vi "GoTo PID rápido.vi"(8 "Position":dbl[](array[numeric]), 11 "Target":dbl[](array[numeric])) -> (3 "Velocity":dbl[](array[numeric]))   [LabVIEW 2016]
uses:
  <vilib>/Analysis/coordinate.llb/2D Cartesian Coordinate Rotation (Scalar).vi
  <vilib>/addons/control/pid/pid.llb/PID (DBL).vi
  <vilib>/addons/control/pid/NI_PID_pid.lvlib
  <vilib>/Analysis/NI_AALPro.lvlib
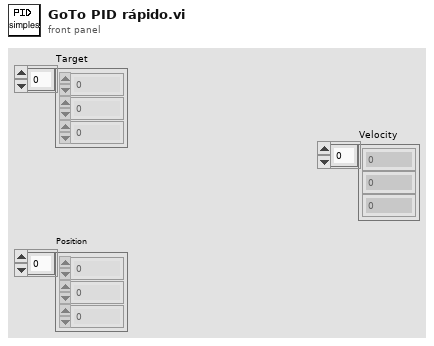
[diagram p1: front panel]
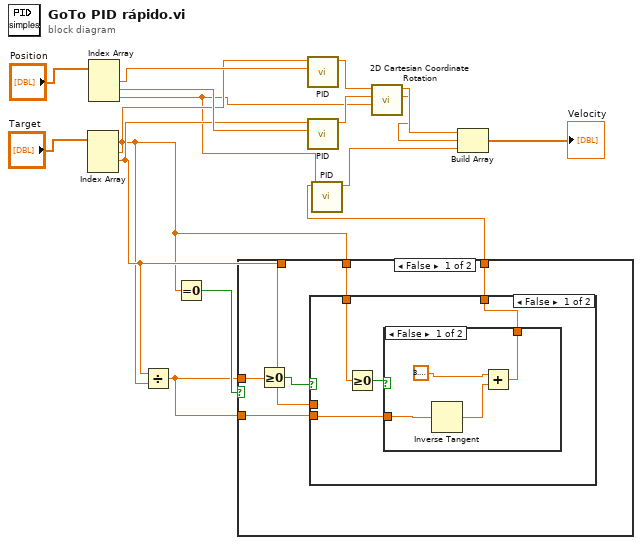
[diagram p0: block diagram]
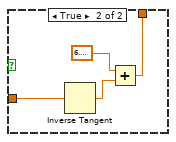
[diagram p2: hidden frame]
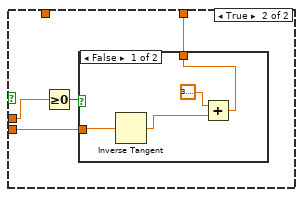
[diagram p3: hidden frame]
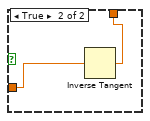
[diagram p4: hidden frame]
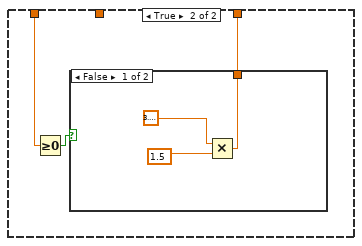
[diagram p5: hidden frame]
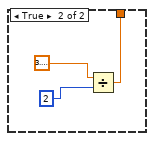
[diagram p6: hidden frame]
diagram:
  n1 = Index Array(array="Target") -> (element #1=w6:dbl, element #2=w8:dbl)  [unwired: 3 in, 1 out]
  n2 = Index Array(array="Position") -> (element #1=w13:dbl, element #2=w12:dbl, element #3=w3:dbl)  [unwired: 3 in]
  n3 = Divide(x=w8, y=w6) -> (x/y=w7:dbl)
  n4 = Equal To 0?(x=w6) -> (x = 0?=w10:bool)
  n5 = case shown="False" w10 {
    tunnel: [w19 w45] -> w9
    tunnel: w7 -> [w22 _]
    tunnel: w8 -> [w20 w47]
    tunnel: w7 -> [w18 _]
    tunnel: w6 -> [w17 _]
    frame False {
      n6 = Greater Or Equal To 0?(x=w22) -> (x >= 0?=w21:bool)
      n7 = case shown="False" w21 {
        tunnel: w20 -> [_ w38]
        tunnel: [w23 w36] -> w19
        tunnel: w18 -> [w24 w35]
        tunnel: w17 -> [w26 _]
        frame False {
          n8 = Greater Or Equal To 0?(x=w26) -> (x >= 0?=w25:bool)
          n9 = case shown="False" w25 {
            tunnel: w24 -> [w30 w34]
            tunnel: [w27 w31] -> w23
            frame False {
              n10 = Inverse Tangent(1:w30) -> (0:w28:dbl)
              n11 = Add(x=3.141592653589793, y=w28) -> (x+y=w27:dbl)
            }
            frame True {
              n12 = Inverse Tangent(1:w34) -> (0:w32:dbl)
              n13 = Add(x=6.283185307179586, y=w32) -> (x+y=w31:dbl)
            }
          }
        }
        frame True {
          n14 = Greater Or Equal To 0?(x=w38) -> (x >= 0?=w37:bool)
          n15 = case shown="False" w37 {
            tunnel: [w40 w43] -> w36
            tunnel: w35 -> [w42 w44]
            frame False {
              n16 = Inverse Tangent(1:w42) -> (0:w41:dbl)
              n17 = Add(x=3.141592653589793, y=w41) -> (x+y=w40:dbl)
            }
            frame True {
              n18 = Inverse Tangent(1:w44) -> (0:w43:dbl)
            }
          }
        }
      }
    }
    frame True {
      n19 = Greater Or Equal To 0?(x=w47) -> (x >= 0?=w46:bool)
      n20 = case shown="False" w46 {
        tunnel: [w49 w52] -> w45
        frame False {
          n21 = Multiply(x=3.141592653589793, y=1.5) -> (x*y=w49:dbl)
        }
        frame True {
          n22 = Divide(x=3.141592653589793, y=2) -> (x/y=w52:dbl)
        }
      }
    }
  }
  n23 = call-poly <vilib>:"PID.vi"("process variable"=w13, "setpoint"=w6) -> ("output"=w5:dbl)  [unwired: 8 in, 1 out]
  n24 = call-poly <vilib>:"PID.vi"("process variable"=w12, "setpoint"=w8) -> ("output"=w4:dbl)  [unwired: 8 in, 1 out]
  n25 = call-poly <vilib>:"PID.vi"("process variable"=w3, "setpoint"=w9) -> ("output"=w11:dbl)  [unwired: 8 in, 1 out]
  n26 = call-poly <vilib>:"2D Cartesian Coordinate Rotation.vi"("theta"=w3, "y"=w4, "x"=w5) -> ("y out"=w1:dbl, "x out"=w2:dbl)  [unwired: 6 in, 1 out]
  n27 = Build Array(w2, w1, w11) -> (→"Velocity":dbl[])
